vi "VIAnUtil Check Type If ErrClust.vi"(8 "error in (no error)":errorcluster, 11 "Data In":variant) -> (0 "error out":errorcluster, 3 "IsErrClust?":bool)   [LabVIEW 2020]
uses:
  Data Type.ctl
  NI_Data Type.lvlib
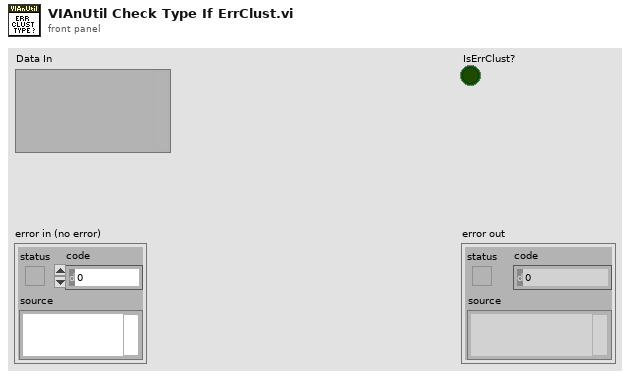
[diagram p1: front panel]
types:
  T1 = typedef "NI_Data Type.lvlib/Data Type.ctl" = enum8{"Invalid Type", "Void", "I8", "I16", "I32", "I64", "U8", "U16", "U32", "U64", "Single Float", "Double Float", "Extended Float", "Single Complex", "Double Complex", "Extended Complex", "Enum U8", "Enum U16", "Enum U32", "Enum U64", "Single Float With Unit", "Double Float With Unit", "Extended Float With Unit", "Single Complex with Unit", "Double Complex with Unit", "Extended Complex with Unit", "Boolean", "String", "Path", "Picture", "Tag", "Array", "Cluster", "Variant", "LV Variant", "Waveform", "Timestamp", "Digital Waveform", "Digital Data", "ExpressData", "Refnum", "External Data", "VI", "Poly VI", "LabVIEW Class Instance", "Fixed Point", "Set Collection", "Map Collection"}
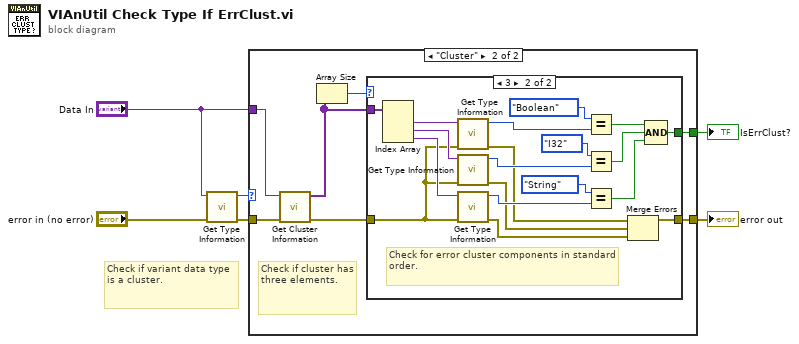
[diagram p0: block diagram]
diagram:
  # "Check if variant data type is a cluster."
  n1 = call "Get Type Information.vi"("error in (no error)"="error in (no error)", "variant"="Data In") -> ("error out"=w3:errorcluster, "type"=w1:T1)  [unwired: 5 in, 3 out]
  n2 = case shown="\"Cluster\"" w1 {
    tunnel: "Data In" -> [_ w14]
    tunnel: [_ w11] -> w6
    tunnel: w3 -> [w7 w10]
    tunnel: [w7 w8] -> w5
    frame Default {
      # "Not a cluster so return false."
    }
    frame "Cluster" {
      # "Check if cluster has three elements."
      n3 = call "Get Cluster Information.vi"("error in (no error)"=w10, "variant"=w14) -> ("error out"=w9:errorcluster, "cluster elements"=w12:variant[])  [unwired: 8 in]
      n4 = Array Size(array=w12) -> (size(s)=w13:i32)
      n5 = case shown="3" w13 {
        tunnel: w12 -> [_ w34]
        tunnel: [_ w30] -> w11
        tunnel: w9 -> [w15 w22]
        tunnel: [w15 w29] -> w8
        frame Default {
          # "Cluster does not have the right number of elements."
        }
        frame 3 {
          # "Check for error cluster components in standard order."
          n6 = Index Array(array=w34) -> (element #1=w20:variant, element #2=w23:variant, element #3=w24:variant)  [unwired: 3 in]
          n7 = call "Get Type Information.vi"("error in (no error)"=w22, "variant"=w20) -> ("error out"=w21:errorcluster, "type"=w19:T1)  [unwired: 5 in, 3 out]
          n8 = call "Get Type Information.vi"("error in (no error)"=w22, "variant"=w23) -> ("error out"=w26:errorcluster, "type"=w25:T1)  [unwired: 5 in, 3 out]
          n9 = call "Get Type Information.vi"("error in (no error)"=w22, "variant"=w24) -> ("error out"=w28:errorcluster, "type"=w27:T1)  [unwired: 5 in, 3 out]
          n10 = Equal?(x=Data_Type."Boolean" ("Type"), y=w19) -> (x = y?=w33:bool)
          n11 = Equal?(x=Data_Type."I32" ("Type"), y=w25) -> (x = y?=w32:bool)
          n12 = Equal?(x=Data_Type."String" ("Type"), y=w27) -> (x = y?=w31:bool)
          n13 = Merge Errors(w21, w26, w28) -> (w29:errorcluster)
          n14 = Compound Arithmetic op=AND(w33, w32, w31) -> (w30:bool)
        }
      }
    }
  }
  "IsErrClust?" <- w6
  "error out" <- w5
